vi "Adjust GPIO T0.vi"(0 "gpio timestamps in":T1(array[cluster])) -> (4 "gpio timestamps out":T1(array[cluster]))   [LabVIEW 2023, in "GettingStarted_Common_148X_Host.lvlib"]
uses:
  GettingStarted_Common_148X_Host.lvlib
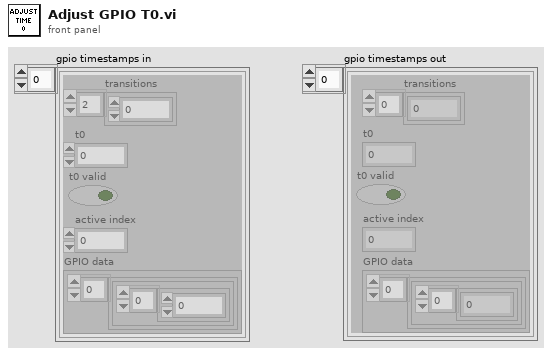
[diagram p1: front panel]
types:
  T1 = cluster{"transitions":u64[], "t0":u64, "t0 valid":bool, "active index":i32, "GPIO data":cluster{cluster{u8[]}[]}}[]
  T2 = cluster{"transitions":u64[], "t0":u64, "t0 valid":bool, "active index":i32, "GPIO data":cluster{cluster{u8[]}[]}}
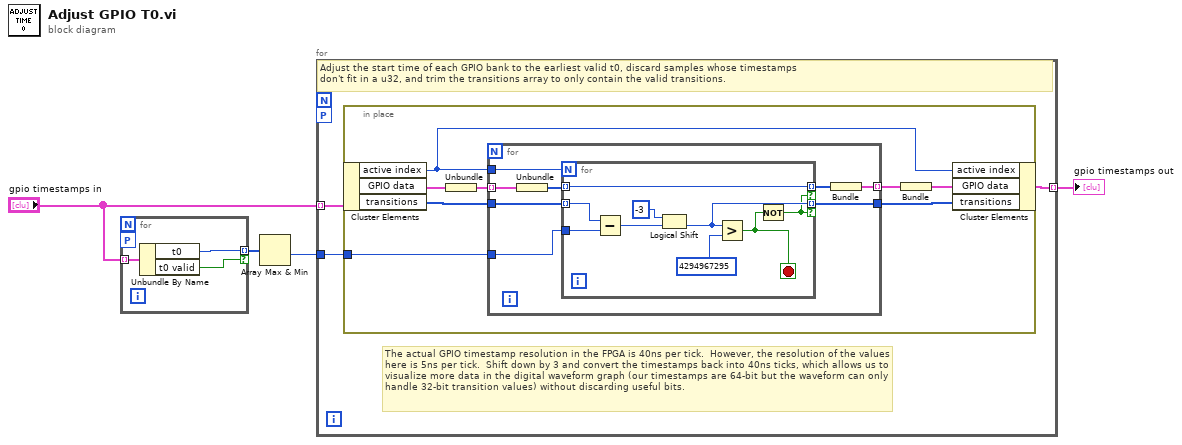
[diagram p0: block diagram]
diagram:
  n1 = for {
    tunnel: "gpio timestamps in" -> [w7] mode=indexing
    tunnel: [w6] -> w1 mode=indexing if=w5
    workers-P: _ -> [_]
    n2 = Unbundle By Name(w7) -> ("t0"=w6:u64, "t0 valid"=w5:bool)
  }
  n3 = Array Max & Min(array=w1) -> (min value=w2:u64)  [unwired: 3 out]
  n4 = for {
    tunnel: w2 -> [w10]
    tunnel: [w8] -> w4 mode=indexing
    tunnel: "gpio timestamps in" -> [w9] mode=indexing
    workers-P: _ -> [_]
    # "The actual GPIO timestamp resolution in the FPGA is 40ns per tick.  However, the resolution of the values here is 5ns per tick.  Shift down by 3 and convert the timestamps back into 40ns ticks, which allows us to visualize more data in the digital waveform graph (our timestamps are 64-bit but the waveform can only handle 32-bit transition values) without discarding useful bits."
    # "Adjust the start time of each GPIO bank to the earliest valid t0, discard samples whose timestamps \ndon't fit in a u32, and trim the transitions array to only contain the valid transitions."
    n5 = in-place {
      in-place-border: w10 -> [w18]
      n6 = in-place-cluster #1(w9) -> ("active index"=w11:i32, "GPIO data"=w15:cluster{cluster{u8[]}[]}, "transitions"=w17:u64[])
      n7 = Unbundle(w15) -> (w14:cluster{u8[]}[])
      n8 = for {
        tunnel: w18 -> [w26]
        tunnel: w17 -> [w25]
        tunnel: [w24] -> w16
        tunnel: w14 -> [w23] mode=indexing
        tunnel: [w19] -> w12 mode=indexing
        tunnel: w11 -> [w21]
        n9 = Unbundle(w23) -> (w20:u8[])
        n10 = for {
          N: w21 -> [_]
          tunnel: [w35] -> w22 mode=indexing if=w27
          tunnel: w20 -> [w35] mode=indexing
          tunnel: w25 -> [w33] mode=indexing
          tunnel: w26 -> [w34]
          tunnel: [w29] -> w24 mode=indexing if=w27
          stop <- w30 stop-if-true
          n11 = Subtract(x=w33, y=w34) -> (x-y=w31:u64)
          n12 = Logical Shift(y=i16 -3, x=w31) -> (x << y=w29:u64)
          n13 = Greater?(x=w29, y=u64 4294967295) -> (0:w30:bool)
          n14 = Not(x=w30) -> (.not. x?=w27:bool)
        }
        n15 = Bundle(w22) -> (w19:cluster{u8[]})  [unwired: 1 in]
      }
      n16 = Bundle(w12) -> (w13:cluster{cluster{u8[]}[]})  [unwired: 1 in]
      n17 = in-place-cluster #1("active index"=w11, "GPIO data"=w13, "transitions"=w16) -> (w8:T2)
    }
  }
  "gpio timestamps out" <- w4
